vi "scan value.vi"() -> ()   [LabVIEW 2017]
panel:
  out "output string":string
  in  "Numeric":dbl
  out "Gauge 2":dbl(knob) scale=0.0..100.0
  out "Gauge":dbl(knob) scale=0.0..10.0
  in  "string":string
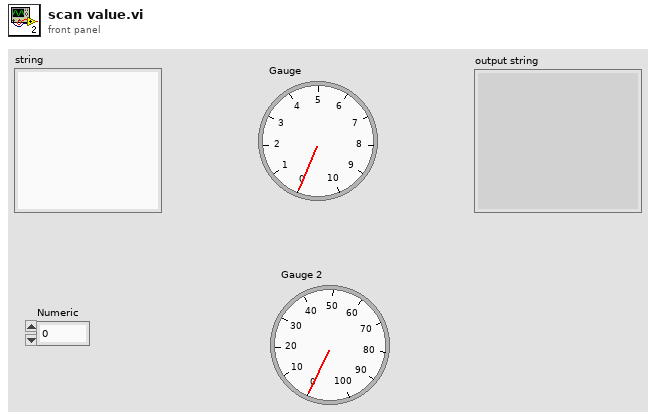
[diagram p1: front panel]
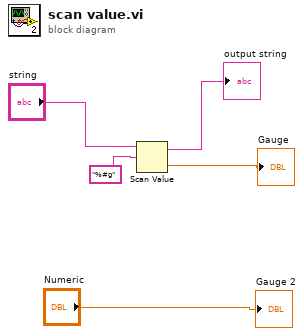
[diagram p0: block diagram]
diagram:
  n1 = Scan Value(string="string", format string="%#g") -> (output string=→"output string":string, value=→"Gauge":dbl)  [unwired: 1 in]
  "Gauge 2" <- "Numeric"
